vi "BDF-Read Record.vi"(0 "Path":path, 5 "Header":T1, 7 "First record":i32, 11 "error in (no error)":errorcluster) -> (15 "error out":errorcluster)   [LabVIEW 2016]
uses:
  BDF-Header.ctl
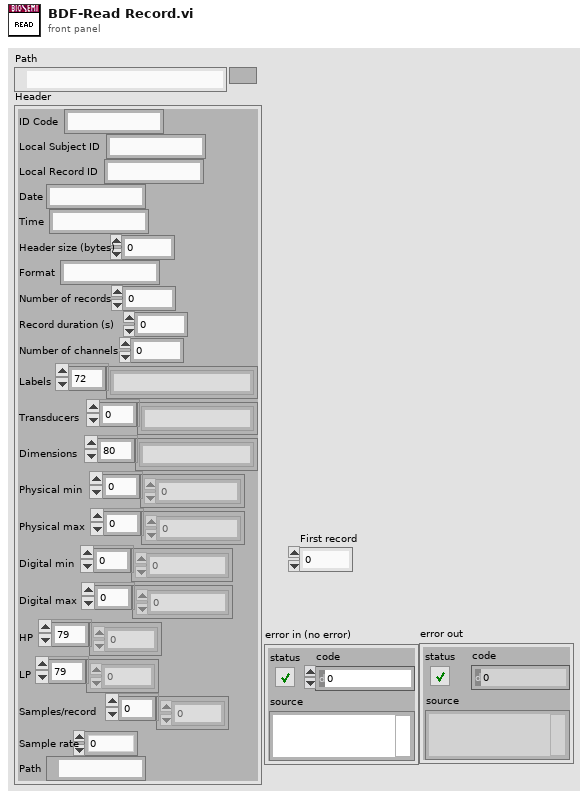
[diagram p1: front panel]
types:
  T1 = typedef "BDF-Header.ctl" = cluster{"ID Code":string, "Local Subject ID":string, "Local Record ID":string, "Date":string, "Time":string, "Header size (bytes)":i32, "Format":string, "Number of records":i32, "Record duration (s)":dbl, "Number of channels":i32, "Labels":string[], "Transducers":string[], "Dimensions":string[], "Physical min":dbl[], "Physical max":dbl[], "Digital min":i32[], "Digital max":i32[], "HP":dbl[], "LP":dbl[], "Samples/record":i32[], "Sample rate":dbl, "Path":path}
  T2 = enum16{"open", "replace", "create", "open or create", "replace or create", "replace or create with confirmation"}
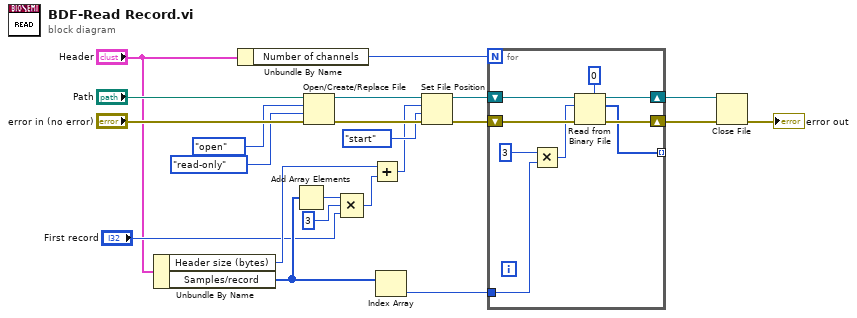
[diagram p0: block diagram]
diagram:
  n1 = Unbundle By Name("Header") -> ("Header size (bytes)"=w10:i32, "Samples/record"=w12:i32[])
  n2 = Unbundle By Name("Header") -> ("Number of channels"=w6:i32)
  n3 = Add Array Elements(numeric array=w12) -> (sum=w11:i32)
  n4 = Open/Create/Replace File(file path (use dialog)="Path", error in="error in (no error)", operation (0:open)=T2."open", access (0:read/write)=enum16{"read/write", "read-only", "write-only"}."read-only") -> (refnum out=w17:refnum<file>, error out=w18:errorcluster)  [unwired: 2 in, 1 out]
  n5 = Compound Arithmetic op=MULTIPLY(w11, 3, "First record") -> (w8:i32)
  n6 = Add(x=w10, y=w8) -> (x+y=w7:i32)
  n7 = Index Array(array=w12) -> (element=w4:i32)  [unwired: 1 in]
  n8 = Set File Position(offset (in bytes) (0)=w7, refnum=w17, from (0:start)=enum16{"start", "end", "current"}."start", error in=w18) -> (refnum out=w14:refnum<file>, error out=w15:errorcluster)
  n9 = for {
    N: w6 -> [_]
    tunnel: w4 -> [w25]
    shift-right: [w26] -> w2
    shift-left: w14 -> [w31]
    shift-right: [w29] -> w1
    shift-left: w15 -> [w30]
    tunnel: [w23] -> _ mode=indexing
    n10 = Multiply(x=3, y=w25) -> (x*y=w27:i32)
    n11 = Read from Binary File(5:u8 0 ("Numeric"), 8:w30, 10:w27, 11:w31) -> (0:w29:errorcluster, 2:w23:u8[], 3:w26:refnum<file>)  [unwired: 2 in, 1 out]
  }
  n12 = Close File(refnum=w2, error in=w1) -> (error out=→"error out":errorcluster)  [unwired: 1 out]
